vi "Hex To Dec.vi"(11 "十六进制字符串":string) -> (0 "32位整型":i32, 1 "字符串":string, 2 "十进制整数":dbl, 3 "十进制整型字符串":string)   [LabVIEW 2014]
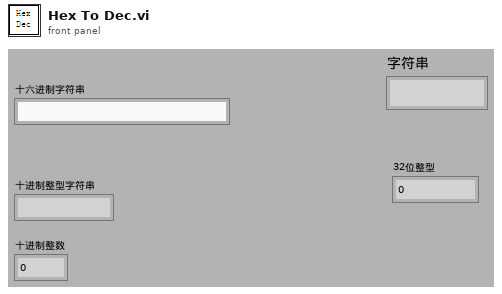
[diagram p1: front panel]
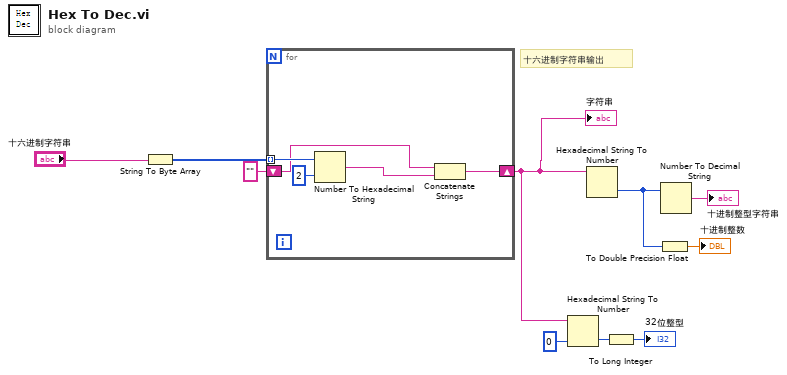
[diagram p0: block diagram]
diagram:
  # "十六进制字符串输出"
  n1 = String To Byte Array(string="十六进制字符串") -> (unsigned byte array=w8:u8[])
  n2 = for {
    tunnel: w8 -> [w15] mode=indexing
    shift-right: [w11] -> w4
    shift-left: "" -> [w14]
    n3 = Number To Hexadecimal String(1:i16 2 ("宽度(-)"), 2:w15) -> (0:w13:string)
    n4 = Concatenate Strings(w14, w13) -> (w11:string)
  }
  "字符串" <- w4
  n5 = Hexadecimal String To Number(string=w4, default (0uL)=i16 0 ("默认(0 U32)")) -> (number=w2:i16)  [unwired: 1 in, 1 out]
  n6 = Hexadecimal String To Number(string=w4) -> (number=w7:u32)  [unwired: 2 in, 1 out]
  n7 = To Long Integer(number=w2) -> (32bit integer=→"32位整型":i32)
  n8 = To Double Precision Float(number=w7) -> (double precision float=→"十进制整数":dbl)
  n9 = Number To Decimal String(number=w7) -> (decimal integer string=→"十进制整型字符串":string)  [unwired: 1 in]
